vi "Get File Versions from PPL VIs.vi"(8 "error in (no error)":errorcluster, 11 "Path":path) -> (0 "error IO":errorcluster, 1 "Table Output":string[](array[string]), 2 "Version String":string, 3 "Version with Hash":string, 4 "Version Cluster":T1)   [LabVIEW 2019]
uses:
  <vilib>/Utility/LVLibp/NI_PackedLibraryUtility.lvlib
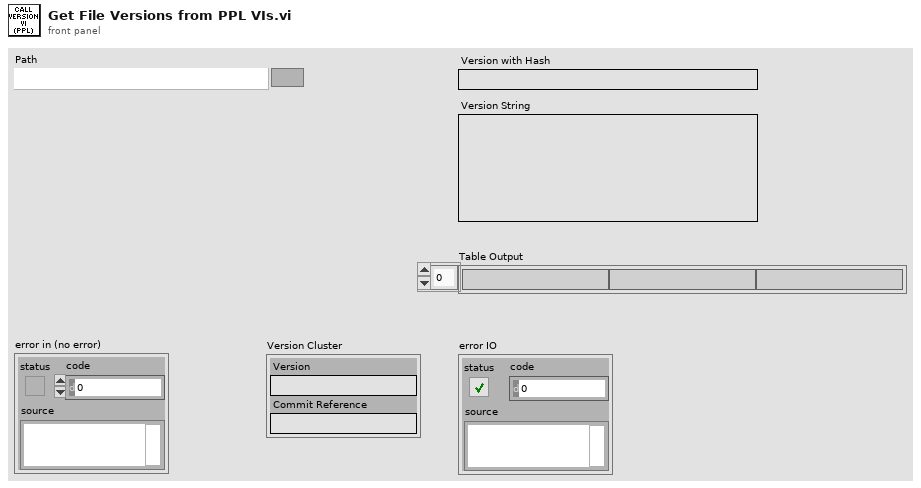
[diagram p1: front panel]
types:
  T1 = cluster{"Version":string, "Commit Reference":string}
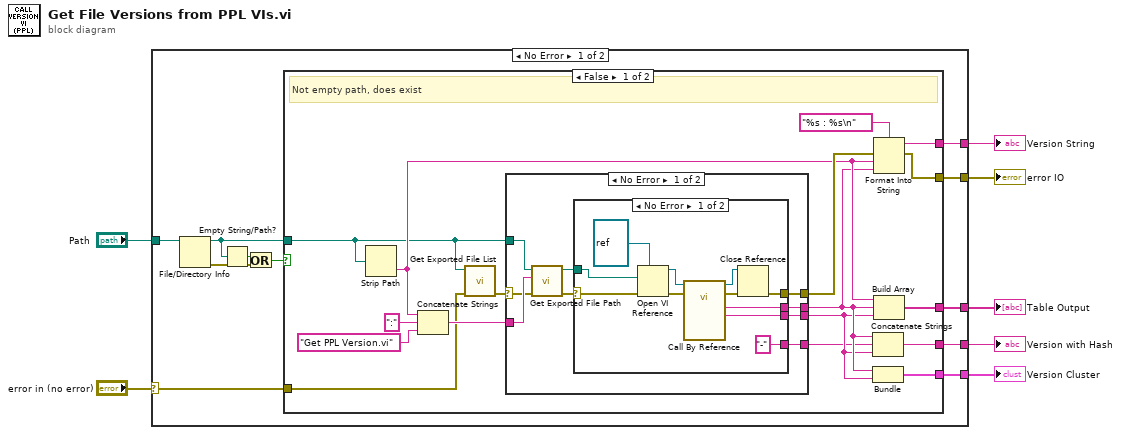
[diagram p0: block diagram]
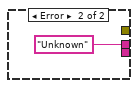
[diagram p2: hidden frame]
diagram:
  n1 = case shown="No Error" "error in (no error)" {
    selector: "error in (no error)" -> [w13 w59]
    tunnel: [w16 _] -> w7
    tunnel: [w18 w59] -> w6
    tunnel: "Path" -> [w12 _]
    tunnel: [w17 _] -> w4
    tunnel: [w15 _] -> w2
    tunnel: [w14 _] -> w1
    frame No Error {
      n2 = File/Directory Info(path=w12) -> (path out=w11:path, error out=w9:errorcluster)  [unwired: 1 in, 5 out]
      n3 = Empty String/Path?(string/path=w11) -> (empty?=w10:bool)
      n4 = Or(x=w10, y=w9) -> (x .or. y?=w8:bool)
      n5 = case shown="False" w8 {
        tunnel: [w35 w58] -> w18
        tunnel: [w28 _] -> w17
        tunnel: [w27 _] -> w16
        tunnel: [w26 _] -> w15
        tunnel: [w23 _] -> w14
        tunnel: w13 -> [w22 w58]
        tunnel: w11 -> [w19 _]
        frame False {
          # "Not empty path, does exist"
          n6 = Strip Path(path=w19) -> (name=w29:string)  [unwired: 1 out]
          n7 = Concatenate Strings(w29, ":" ("string"), "Get PPL Version.vi" ("qualified name")) -> (w33:string)
          n8 = call <vilib>:"Get Exported File List.vi"("error in (no error)"=w22, "packed library path"=w19) -> ("error out"=w21:errorcluster)  [unwired: 7 in, 2 out]
          n9 = case shown="No Error" w21 {
            selector: w21 -> [w37 w57]
            tunnel: w33 -> [w44 _]
            tunnel: [w42 w57] -> w30
            tunnel: [w40 _] -> w25
            tunnel: [w39 _] -> w24
            tunnel: w19 -> [w38 _]
            tunnel: [w36 _] -> w20
            frame No Error {
              n10 = call <vilib>:"Get Exported File Path.vi"("error in (no error)"=w37, "qualified name"=w44, "packed library path"=w38) -> ("error out"=w41:errorcluster, "path"=w43:path)  [unwired: 7 in]
              n11 = case shown="No Error" w41 {
                selector: w41 -> [w47 _]
                tunnel: w43 -> [w55 _]
                tunnel: [w51 "Unknown" ("Version")] -> w40
                tunnel: [w49 _] -> w42
                tunnel: [w46 _] -> w39
                tunnel: ["-" ("string") _] -> w36
                frame No Error {
                  n12 = Open VI Reference(type specifier VI Refnum (for type only)=refnum<vi> refnum, vi path=w55, error in (no error)=w47) -> (vi reference=w53:refnum<vi>, error out=w54:errorcluster)  [unwired: 3 in]
                  n13 = call-by-ref "?"(reference=w53, error in=w54) -> (reference out=w48:refnum<vi>, error out=w50:errorcluster, "Commit Reference"=w46:string, "Version"=w51:string)  [unwired: 10 in]
                  n14 = Close Reference(reference=w48, error in (no error)=w50) -> (error out=w49:errorcluster)
                }
                frame Error {
                }
              }
            }
            frame Error {
              # "Not a PPL file"
            }
          }
          n15 = Concatenate Strings(w25, w20, w24) -> (w26:string)
          n16 = Bundle("Version"=w25, "Commit Reference"=w24) -> (w23:T1)  [unwired: 1 in]
          n17 = Format Into String(format string="%s : %s\n", error in=w30, w29, w25) -> (resulting string=w27:string, error out=w35:errorcluster)  [unwired: 1 in]
          n18 = Build Array(w29, w25, w24) -> (w28:string[])
        }
        frame True {
        }
      }
    }
    frame Error {
    }
  }
  "Version String" <- w7
  "error IO" <- w6
  "Table Output" <- w4
  "Version with Hash" <- w2
  "Version Cluster" <- w1
